vi "main.vi"() -> ()   [LabVIEW 2018]
uses:
  enums.ctl
  Consumer_Data.ctl
panel:
  out "CUSTOMER":string
  in  "Run":bool
  out "Final Weight":dbl
  in  "Home Button":bool
  in  "Continue":bool
  out "State":T1
  in  "Emergency Stop":bool=TRUE
  out "return value":string
  in  "Edit Thresholds":bool
  in  "Update Variant Program":bool
  out "Total Lines":string
  in  "error in (no error)":errorcluster
  in  "Verify Button":bool
  in  "SERIAL NUMBER":string
  out "error out":errorcluster
  # "GAPFILLER WEIGHT"
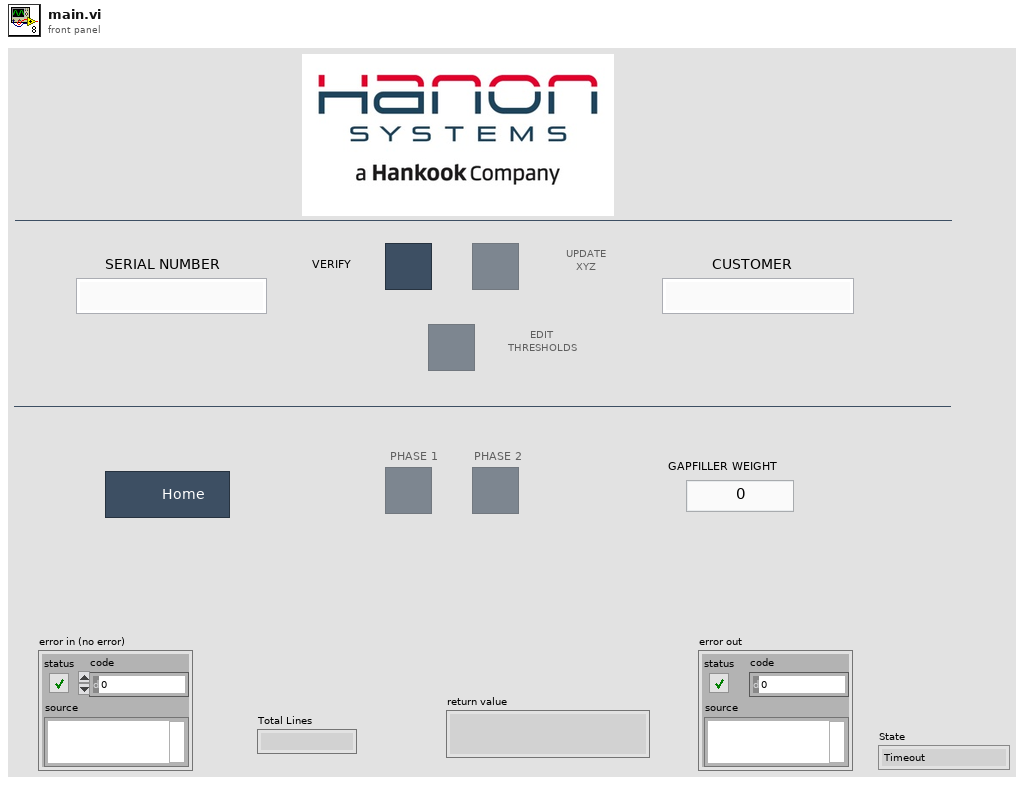
[diagram p1: front panel]
types:
  T1 = typedef "enums.ctl" = enum16{"Timeout", "Init", "Verify", "Update Variant", "Run", "Continue", "Edit Thresholds", "Home", "Exit"}
  T2 = typedef "Consumer_Data.ctl" = cluster{"Customer Variant":string, "Total Lines":string, "include path":path}
  T3 = enum8{"Enabled", "Disabled", "Disabled and Grayed Out"}
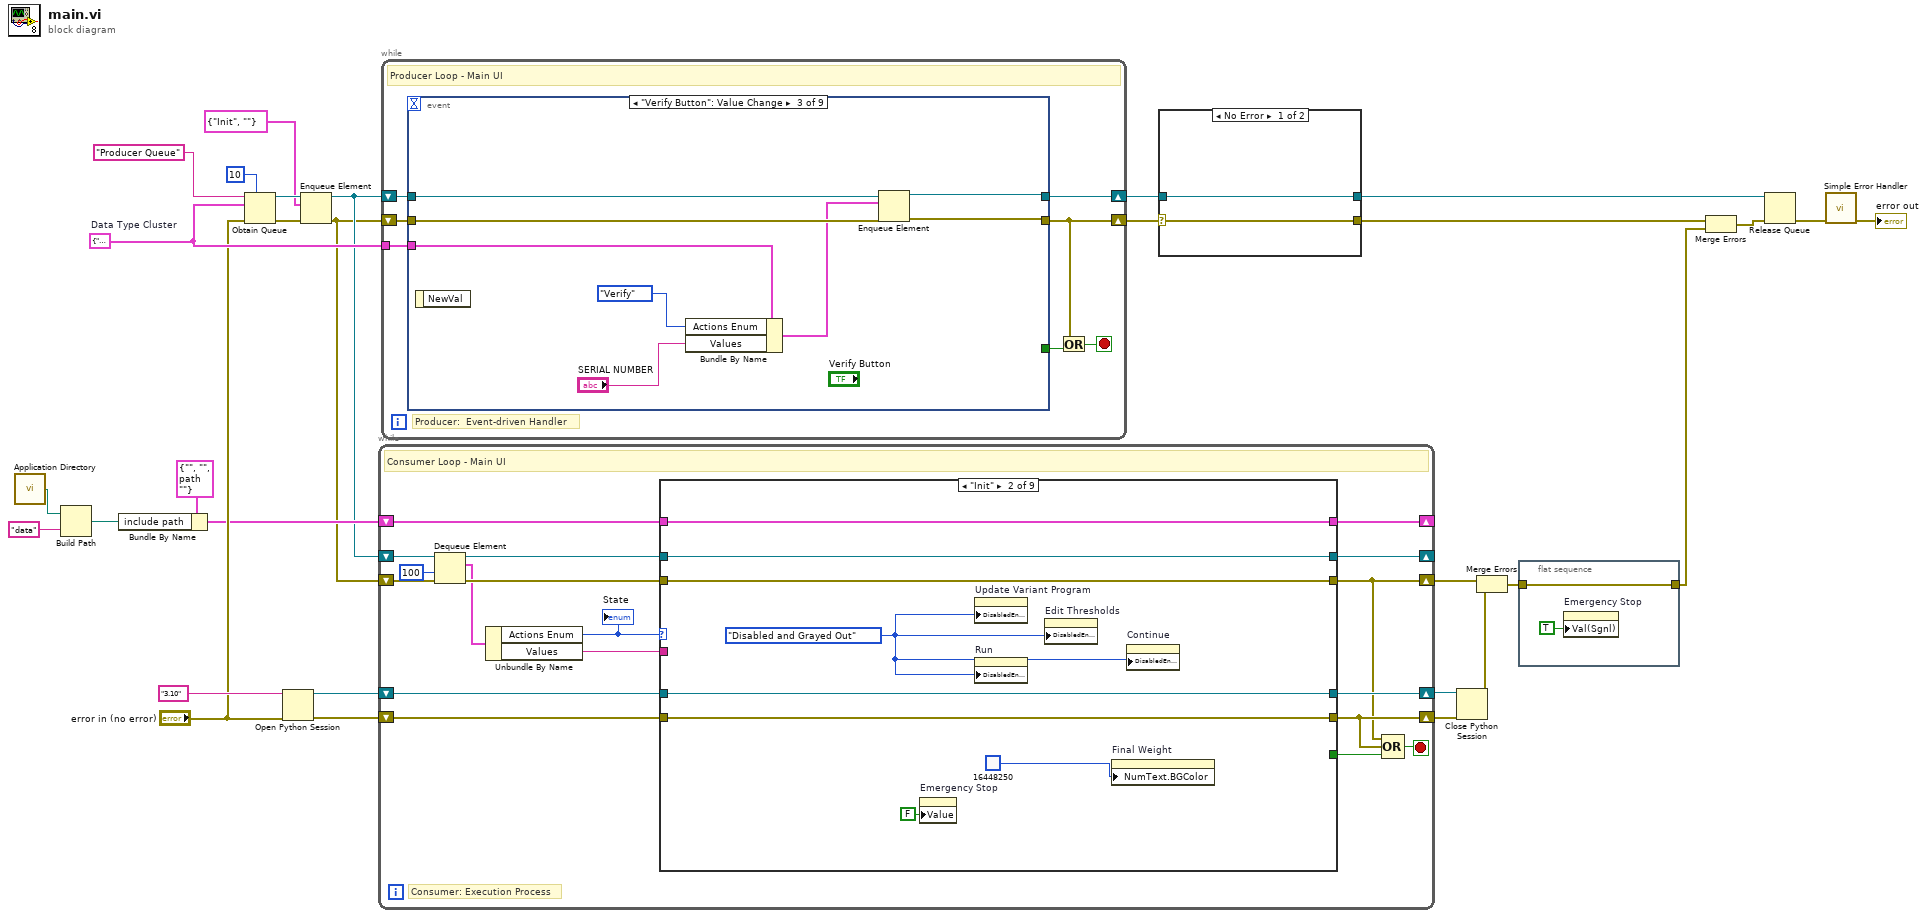
[diagram p0: block diagram]
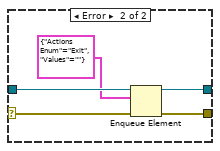
[diagram p2: hidden frame]
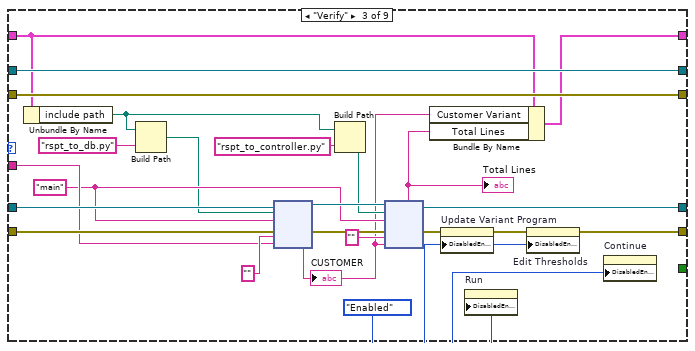
[diagram p4: hidden frame]
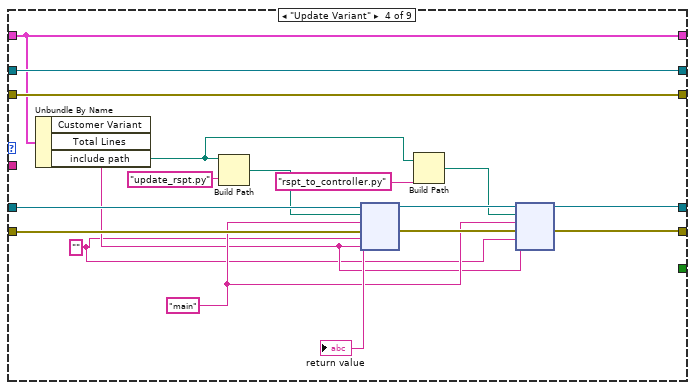
[diagram p5: hidden frame]
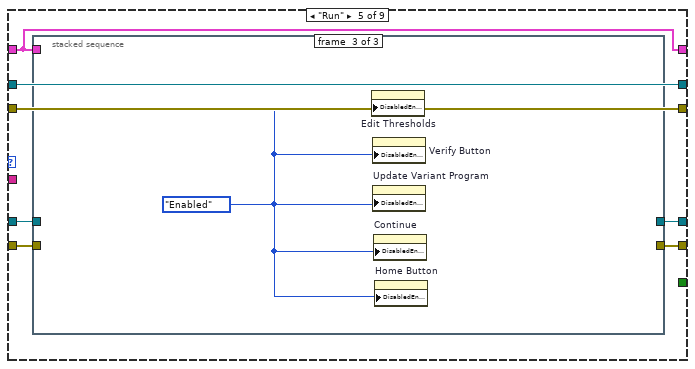
[diagram p6: hidden frame]
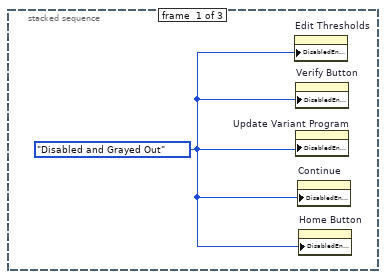
[diagram p7: hidden frame]
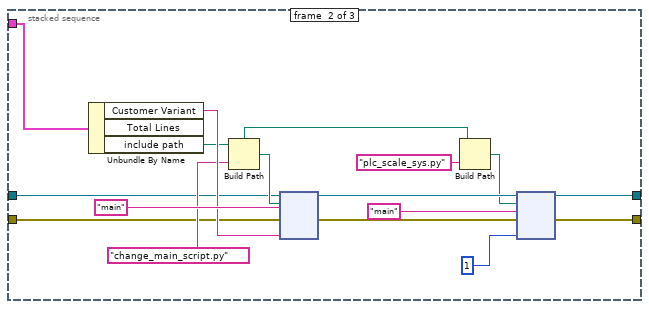
[diagram p8: hidden frame]
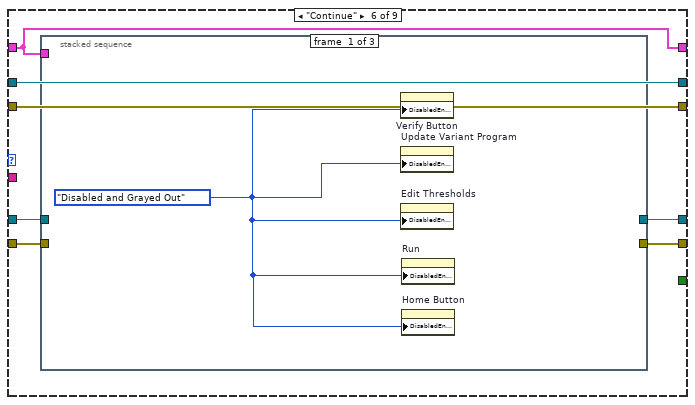
[diagram p9: hidden frame]
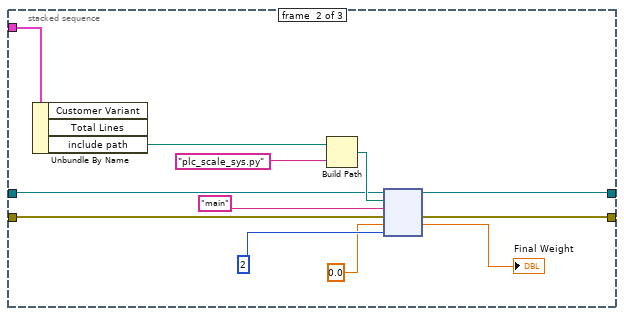
[diagram p10: hidden frame]
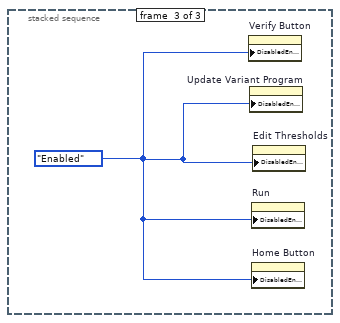
[diagram p11: hidden frame]
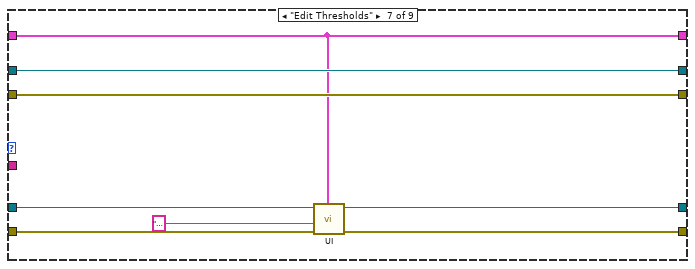
[diagram p12: hidden frame]
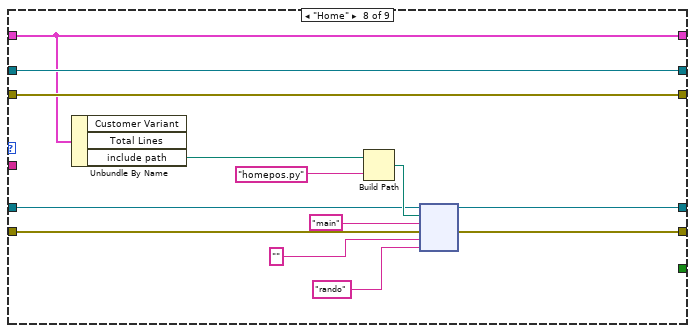
[diagram p13: hidden frame]
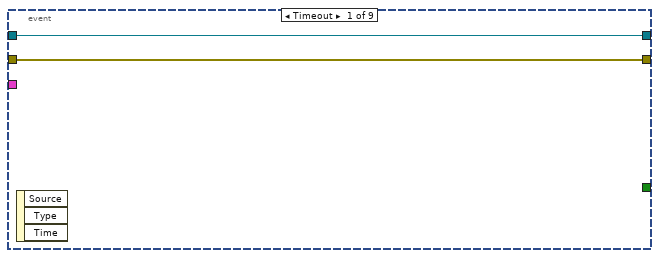
[diagram p15: hidden frame]
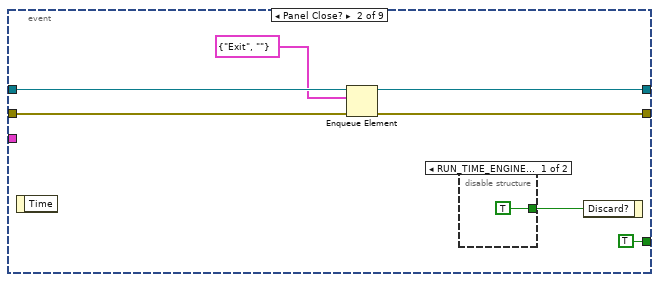
[diagram p16: hidden frame]
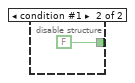
[diagram p17: hidden frame]
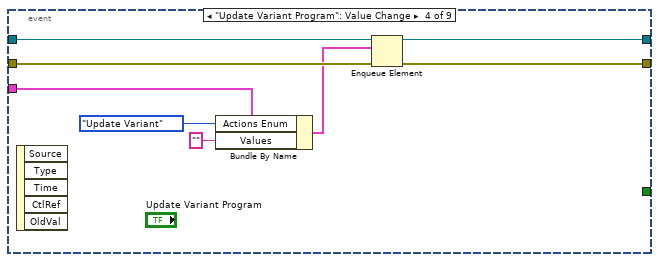
[diagram p18: hidden frame]
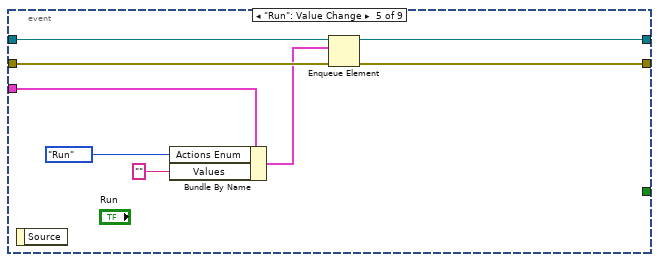
[diagram p19: hidden frame]
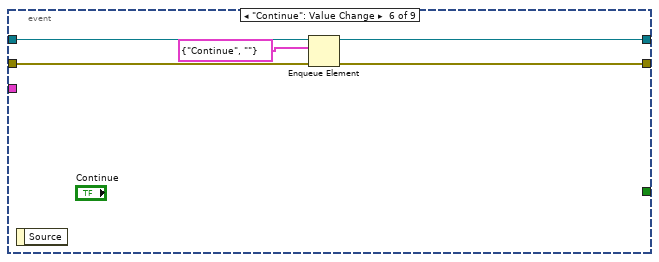
[diagram p20: hidden frame]
diagram:
  w27 = cluster{"Actions Enum":T1, "Values":string} {"Actions Enum"=enum."Timeout", "Values"=""}  # Data Type Cluster
  n1 = call <vilib>:"Application Directory.vi"() -> ("Application Directory"=w20:path)
  n2 = Build Path(base path=w20, name or relative path="data") -> (appended path=w16:path)
  n3 = Bundle By Name(cluster=T2 {"Customer Variant"="", "Total Lines"="", "include path"=path ""} ("Consumer Data"), "include path"=w16) -> (w17:T2)
  n4 = Obtain Queue(max queue size (-1, unlimited)=10, name (unnamed)="Producer Queue", element data type=w27, error in (no error)="error in (no error)") -> (queue out=w15:refnum<queue>, error out=w13:errorcluster)  [unwired: 1 in, 1 out]
  n5 = Open Python Session(python version="3.10" ("Python version"), 3:"error in (no error)") -> (session out=w25:refnum<k35>, error out=w24:errorcluster)  [unwired: 1 in]
  n6 = Enqueue Element(queue=w15, element=cluster{T1, string} {enum."Init", ""}, error in (no error)=w13) -> (queue out=w14:refnum<queue>, error out=w12:errorcluster)  [unwired: 1 in, 1 out]
  n7 = while {
    shift-right: [w32] -> w5
    shift-left: w12 -> [w47]
    shift-right: [w43] -> _
    shift-left: w14 -> [w42]
    shift-right: [w37] -> w23
    shift-left: w25 -> [w36]
    shift-right: [w33] -> w22
    shift-left: w24 -> [w35]
    shift-right: [w38] -> _
    shift-left: w17 -> [w39]
    stop <- w34 stop-if-true
    # "Consumer: Execution Process"
    # "Consumer Loop - Main UI"
    n8 = Dequeue Element(queue=w42, timeout in ms (-1)=100, error in (no error)=w47) -> (queue out=w45:refnum<queue>, element=w41:cluster{"Actions Enum":T1, "Values":string}, error out=w46:errorcluster)  [unwired: 1 out]
    n9 = Unbundle By Name(w41) -> ("Actions Enum"=w31:T1, "Values"=w40:string)
    "State" <- w31
    n10 = case shown="\"Init\"" w31 {
      tunnel: w46 -> [w53 w61 w84 w102 w109 w134 w156 w169 w175]
      tunnel: [w53 w61 w84 w102 w109 w134 w156 w169 w175] -> w32
      tunnel: w45 -> [w52 w60 w83 w101 w108 w133 w155 w168 w174]
      tunnel: [w52 w60 w83 w101 w108 w133 w155 w168 w174] -> w43
      tunnel: [_ _ _ _ _ _ _ _ TRUE] -> w44
      tunnel: w40 -> [_ _ w79 _ _ _ _ _ _]
      tunnel: w36 -> [w51 w59 w82 w100 w107 w132 w152 w162 w172]
      tunnel: [w51 w59 w77 w93 w105 w131 w151 w161 w172] -> w37
      tunnel: w35 -> [w50 w58 w81 w99 w106 w129 w154 w160 w171]
      tunnel: [w50 w58 w64 w91 w104 w130 w150 w159 w171] -> w33
      tunnel: [w49 w57 w74 w98 w103 w128 w149 w163 w170] -> w38
      tunnel: w39 -> [w49 w57 w72 w98 w103 w128 w149 w163 w170]
      frame "Timeout", Default {
      }
      frame "Init" {
        w55 = T3."Disabled and Grayed Out" ("Disabled")
        n11 = property on="Emergency Stop" class="Bool (strict)"("Value"=FALSE ("Emergency_Stop")) -> ()  [unwired: 2 in, 2 out]
        n12 = property on="Update Variant Program" class="Bool"("DisabledEnum"=w55) -> ()  [unwired: 2 in, 2 out]
        n13 = property on="Run" class="Bool"("DisabledEnum"=w55) -> ()  [unwired: 2 in, 2 out]
        n14 = property on="Edit Thresholds" class="Bool"("DisabledEnum"=w55) -> ()  [unwired: 2 in, 2 out]
        n15 = property on="Final Weight" class="DigNum (strict)"("NumText.BGColor"=u32 16448250) -> ()  [unwired: 2 in, 2 out]
        n16 = property on="Continue" class="Bool"("DisabledEnum"=w55) -> ()  [unwired: 2 in, 2 out]
      }
      frame "Verify" {
        w63 = T3."Enabled" ("Disabled")
        w76 = "main" ("function name")
        n17 = Unbundle By Name(w72) -> ("include path"=w68:path)
        n18 = Build Path(base path=w68, name or relative path="rspt_to_db.py") -> (appended path=w70:path)
        n19 = node(w82, w70, w76, w81, "", w79) -> (w78:refnum<k35>, w66:errorcluster, w62:string)  [unwired: 1 in, 2 out]
        "CUSTOMER" <- w62
        n20 = Build Path(base path=w68, name or relative path="rspt_to_controller.py") -> (appended path=w67:path)
        n21 = node(w78, w67, w76, "", w62) -> (w77:refnum<k35>, w73:string)  [unwired: 2 in, 3 out]
        "Total Lines" <- w73
        n22 = Bundle By Name(cluster=w72, "Customer Variant"=w62, "Total Lines"=w73) -> (w74:T2)
        n23 = property on="Update Variant Program" class="Bool"(error in=w66, "DisabledEnum"=w63) -> (error out=w65:errorcluster)  [unwired: 1 in, 1 out]
        n24 = property on="Run" class="Bool"("DisabledEnum"=w63) -> ()  [unwired: 2 in, 2 out]
        n25 = property on="Edit Thresholds" class="Bool"(error in=w65, "DisabledEnum"=w63) -> (error out=w64:errorcluster)  [unwired: 1 in, 1 out]
        n26 = property on="Continue" class="Bool"("DisabledEnum"=w63) -> ()  [unwired: 2 in, 2 out]
      }
      frame "Update Variant" {
        w85 = ""
        w90 = "main" ("function name")
        n27 = Unbundle By Name(w98) -> ("Customer Variant"=w86:string, "include path"=w88:path)  [unwired: 1 out]
        n28 = Build Path(base path=w88, name or relative path="update_rspt.py") -> (appended path=w95:path)
        n29 = node(w100, w95, w90, w99, w85, w86) -> (w94:refnum<k35>, w92:errorcluster, →"return value":string)  [unwired: 1 in, 2 out]
        n30 = Build Path(base path=w88, name or relative path="rspt_to_controller.py") -> (appended path=w89:path)
        n31 = node(w94, w89, w90, w92, w85, w86) -> (w93:refnum<k35>, w91:errorcluster)  [unwired: 2 in, 2 out]
      }
      frame "Run" {
        n32 = stacked-sequence {
          tunnel: w107 -> [_ w122 _]
          tunnel: w106 -> [_ w121 _]
          tunnel: [_ w111 _] -> w105
          tunnel: [_ w118 _] -> w104
          tunnel: w103 -> [_ w113 _]
          frame #0 {
            w110 = T3."Disabled and Grayed Out" ("Disabled")
            n33 = property on="Edit Thresholds" class="Bool"("DisabledEnum"=w110) -> ()  [unwired: 2 in, 2 out]
            n34 = property on="Verify Button" class="Bool"("DisabledEnum"=w110) -> ()  [unwired: 2 in, 2 out]
            n35 = property on="Update Variant Program" class="Bool"("DisabledEnum"=w110) -> ()  [unwired: 2 in, 2 out]
            n36 = property on="Continue" class="Bool"("DisabledEnum"=w110) -> ()  [unwired: 2 in, 2 out]
            n37 = property on="Home Button" class="Bool"("DisabledEnum"=w110) -> ()  [unwired: 2 in, 2 out]
          }
          frame #1 {
            n38 = Unbundle By Name(w113) -> ("Customer Variant"=w125:string, "include path"=w114:path)  [unwired: 1 out]
            n39 = Build Path(base path=w114, name or relative path="change_main_script.py") -> (appended path=w123:path)
            n40 = node(w122, w123, "main" ("function name"), w121, w125) -> (w120:refnum<k35>, w119:errorcluster)  [unwired: 3 in, 2 out]
            n41 = Build Path(base path=w114, name or relative path="plc_scale_sys.py") -> (appended path=w117:path)
            n42 = node(w120, w117, "main" ("function name"), w119, 1) -> (w111:refnum<k35>, w118:errorcluster)  [unwired: 3 in, 2 out]
          }
          frame #2 {
            w127 = T3."Enabled" ("Disabled")
            n43 = property on="Edit Thresholds" class="Bool"("DisabledEnum"=w127) -> ()  [unwired: 2 in, 2 out]
            n44 = property on="Verify Button" class="Bool"("DisabledEnum"=w127) -> ()  [unwired: 2 in, 2 out]
            n45 = property on="Update Variant Program" class="Bool"("DisabledEnum"=w127) -> ()  [unwired: 2 in, 2 out]
            n46 = property on="Continue" class="Bool"("DisabledEnum"=w127) -> ()  [unwired: 2 in, 2 out]
            n47 = property on="Home Button" class="Bool"("DisabledEnum"=w127) -> ()  [unwired: 2 in, 2 out]
          }
        }
      }
      frame "Continue" {
        n48 = stacked-sequence {
          tunnel: w132 -> [_ w146 _]
          tunnel: [_ w145 _] -> w131
          tunnel: [_ w144 _] -> w130
          tunnel: w129 -> [_ w143 _]
          tunnel: w128 -> [_ w142 _]
          frame #0 {
            w135 = T3."Disabled and Grayed Out" ("Disabled")
            n49 = property on="Verify Button" class="Bool"("DisabledEnum"=w135) -> ()  [unwired: 2 in, 2 out]
            n50 = property on="Update Variant Program" class="Bool"("DisabledEnum"=w135) -> ()  [unwired: 2 in, 2 out]
            n51 = property on="Edit Thresholds" class="Bool"("DisabledEnum"=w135) -> ()  [unwired: 2 in, 2 out]
            n52 = property on="Run" class="Bool"("DisabledEnum"=w135) -> ()  [unwired: 2 in, 2 out]
            n53 = property on="Home Button" class="Bool"("DisabledEnum"=w135) -> ()  [unwired: 2 in, 2 out]
          }
          frame #1 {
            n54 = Unbundle By Name(w142) -> ("include path"=w141:path)  [unwired: 2 out]
            n55 = Build Path(base path=w141, name or relative path="plc_scale_sys.py") -> (appended path=w147:path)
            n56 = node(w146, w147, "main" ("function name"), w143, 0.0, 2) -> (w145:refnum<k35>, w144:errorcluster, →"Final Weight":dbl)  [unwired: 1 in, 2 out]
          }
          frame #2 {
            w148 = T3."Enabled" ("Disabled")
            n57 = property on="Verify Button" class="Bool"("DisabledEnum"=w148) -> ()  [unwired: 2 in, 2 out]
            n58 = property on="Update Variant Program" class="Bool"("DisabledEnum"=w148) -> ()  [unwired: 2 in, 2 out]
            n59 = property on="Run" class="Bool"("DisabledEnum"=w148) -> ()  [unwired: 2 in, 2 out]
            n60 = property on="Home Button" class="Bool"("DisabledEnum"=w148) -> ()  [unwired: 2 in, 2 out]
            n61 = property on="Edit Thresholds" class="Bool"("DisabledEnum"=w148) -> ()  [unwired: 2 in, 2 out]
          }
        }
      }
      frame "Edit Thresholds" {
        n62 = call "UI.vi"("Consumer Data"=w149, "error in (no error)"=w154, "function name"="main", "session in"=w152) -> ("error out"=w150:errorcluster, "session out"=w151:refnum<k35>)  [unwired: 6 in]
      }
      frame "Home" {
        n63 = Unbundle By Name(w163) -> ("include path"=w166:path)  [unwired: 2 out]
        n64 = Build Path(base path=w166, name or relative path="homepos.py") -> (appended path=w167:path)
        n65 = node(w162, w167, "main" ("function name"), w160, "", "rando") -> (w161:refnum<k35>, w159:errorcluster)  [unwired: 2 in, 2 out]
      }
      frame "Exit" {
      }
    }
    n66 = Compound Arithmetic op=OR(w32, w33, w44) -> (w34:bool)
  }
  n67 = while {
    shift-right: [w181] -> w9
    shift-left: w14 -> [w182]
    shift-right: [w176] -> w10
    shift-left: w12 -> [w180]
    tunnel: w27 -> [w178]
    stop <- w177 stop-if-true
    # "Producer:  Event-driven Handler"
    # "Producer Loop - Main UI"
    n68 = event shown="[2] \"Verify Button\": Value Change" {
      selector: _ -> [_ _ _ _ _ _ _ _ _]
      dyn-events: _ -> [_ _ _ _ _ _ _ _ _]
      timeout: _ -> [_ _ _ _ _ _ _ _ _]
      tunnel: w182 -> [w184 w191 w201 w207 w216 w222 w226 w233 w239]
      tunnel: [w184 w190 w200 w208 w217 w221 w227 w233 w238] -> w181
      tunnel: w180 -> [w183 w189 w199 w205 w215 w220 w225 w232 w241]
      tunnel: [w183 w188 w198 w206 w214 w219 w224 w232 w240] -> w176
      tunnel: [_ TRUE ("Discard?") _ _ _ _ _ TRUE ("Discard?") _] -> w179
      tunnel: w178 -> [_ _ w195 w204 w211 _ w228 _ w234]
      event Timeout {
        n69 = event-data() -> ()  [unwired: 1 in, 3 out]
      }
      event Panel Close? {
        n70 = event-data() -> ()  [unwired: 1 in, 1 out]
        n71 = Enqueue Element(queue=w191, element=cluster{T1, string} {enum."Exit", ""}, error in (no error)=w189) -> (queue out=w190:refnum<queue>, error out=w188:errorcluster)  [unwired: 1 in, 1 out]
        n72 = disable-structure shown="RUN_TIME_ENGINE==False" {
          disable-tunnel: [TRUE ("Discard?") FALSE ("Discard?")] -> w185
          frame condition #0 (active) {
          }
          frame condition #1 {
          }
        }
        n73 = event-data("Discard?"=w185) -> ()  [unwired: 1 in, 1 out]
      }
      event "Verify Button": Value Change {
        n74 = event-data() -> ()  [unwired: 1 in, 1 out]
        n75 = Bundle By Name(cluster=w195, "Actions Enum"=enums."Verify", "Values"="SERIAL NUMBER") -> (w196:cluster{"Actions Enum":T1, "Values":string})
        n76 = Enqueue Element(queue=w201, element=w196, error in (no error)=w199) -> (queue out=w200:refnum<queue>, error out=w198:errorcluster)  [unwired: 1 in, 1 out]
      }
      event "Update Variant Program": Value Change {
        n77 = event-data() -> ()  [unwired: 1 in, 5 out]
        n78 = Bundle By Name(cluster=w204, "Actions Enum"=enums."Update Variant", "Values"="") -> (w203:cluster{"Actions Enum":T1, "Values":string})
        n79 = Enqueue Element(queue=w207, element=w203, error in (no error)=w205) -> (queue out=w208:refnum<queue>, error out=w206:errorcluster)  [unwired: 1 in, 1 out]
      }
      event "Run": Value Change {
        n80 = event-data() -> ()  [unwired: 1 in, 1 out]
        n81 = Bundle By Name(cluster=w211, "Actions Enum"=enums."Run", "Values"="") -> (w210:cluster{"Actions Enum":T1, "Values":string})
        n82 = Enqueue Element(queue=w216, element=w210, error in (no error)=w215) -> (queue out=w217:refnum<queue>, error out=w214:errorcluster)  [unwired: 1 in, 1 out]
      }
      event "Continue": Value Change {
        n83 = event-data() -> ()  [unwired: 1 in, 1 out]
        n84 = Enqueue Element(queue=w222, element=cluster{T1, string} {enum."Continue", ""}, error in (no error)=w220) -> (queue out=w221:refnum<queue>, error out=w219:errorcluster)  [unwired: 1 in, 1 out]
      }
      event "Edit Thresholds": Value Change {
        n85 = event-data() -> ()  [unwired: 1 in, 3 out]
        n86 = Bundle By Name(cluster=w228, "Actions Enum"=enums."Edit Thresholds", "Values"="") -> (w229:cluster{"Actions Enum":T1, "Values":string})
        n87 = Enqueue Element(queue=w226, element=w229, error in (no error)=w225) -> (queue out=w227:refnum<queue>, error out=w224:errorcluster)  [unwired: 1 in, 1 out]
      }
      event "Emergency Stop": Value Change {
        n88 = event-data() -> ()  [unwired: 1 in, 5 out]
      }
      event "Home Button": Value Change {
        n89 = event-data() -> ()  [unwired: 1 in, 5 out]
        n90 = Bundle By Name(cluster=w234, "Actions Enum"=enums."Home", "Values"="") -> (w235:cluster{"Actions Enum":T1, "Values":string})
        n91 = Enqueue Element(queue=w239, element=w235, error in (no error)=w241) -> (queue out=w238:refnum<queue>, error out=w240:errorcluster)  [unwired: 1 in, 1 out]
      }
    }
    n92 = Or(x=w176, y=w179) -> (x .or. y?=w177:bool)
  }
  n93 = case shown="No Error" w10 {
    selector: w10 -> [w242 w248]
    tunnel: w9 -> [w243 w247]
    tunnel: [w243 w246] -> w8
    tunnel: [w242 w245] -> w7
    frame No Error {
    }
    frame Error {
      n94 = Enqueue Element(queue=w247, element=cluster{"Actions Enum":T1, "Values":string} {"Actions Enum"=enum."Exit", "Values"=""}, error in (no error)=w248) -> (queue out=w246:refnum<queue>, error out=w245:errorcluster)  [unwired: 1 in, 1 out]
    }
  }
  n95 = Close Python Session(session in=w23, error in=w22) -> (11:w4:errorcluster)
  n96 = Merge Errors(w5, w4) -> (w3:errorcluster)
  n97 = flat-sequence {
    tunnel: w3 -> [w249]
    tunnel: [w249] -> w2
    frame #0 {
      n98 = property on="Emergency Stop" class="Bool (strict)"("Val(Sgnl)"=TRUE ("Value (Signaling)")) -> ()  [unwired: 2 in, 2 out]
    }
  }
  n99 = Merge Errors(w7, w2) -> (w6:errorcluster)
  n100 = Release Queue(queue=w8, error in (no error)=w6) -> (error out=w29:errorcluster)  [unwired: 1 in, 2 out]
  n101 = call <vilib>:"Simple Error Handler.vi"("error in (no error)"=w29) -> ("error out"=→"error out":errorcluster)  [unwired: 4 in, 4 out]
